vi "Write Mode.vi"(10 "Mode":string, 11 "Motor Configuration in":refnum<class "Motor Configuration.lvclass">) -> (3 "Motor Configuration out":refnum<class "Motor Configuration.lvclass">)   [LabVIEW 2016, in "Hardware.lvlib" / "Motor.lvlib" / "Motor Configuration.lvclass"]
uses:
  <userlib>/Common Components/Hardware/Motor/Motor Config/Motor Configuration.lvclass
  <userlib>/Common Components/Hardware/Motor/Motor Config/Motor Configuration.lvclass/Motor Configuration.ctl
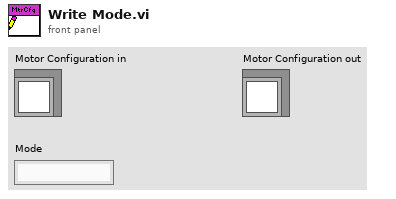
[diagram p1: front panel]
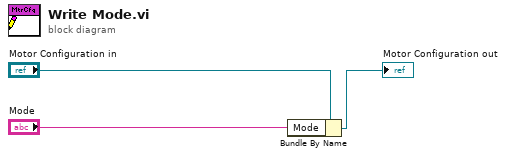
[diagram p0: block diagram]
diagram:
  n1 = Bundle By Name(cluster="Motor Configuration in", "Mode"="Mode") -> (→"Motor Configuration out":refnum<class "Motor Configuration.lvclass">)
